vi "Modbus_Get_Temp.vi"(10 "register values":u16[](array[numeric]), 11 "Temp. unit:":u16) -> (2 "Numeric":dbl, 3 "Strings []":string[](array[string]))   [LabVIEW 2020]
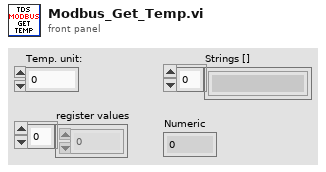
[diagram p1: front panel]
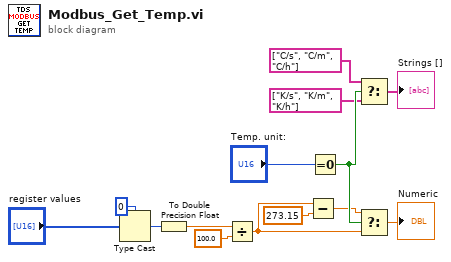
[diagram p0: block diagram]
diagram:
  n1 = Type Cast(type=0, x="register values") -> (*(type *) &x=w2:i32)
  n2 = To Double Precision Float(number=w2) -> (double precision float=w4:dbl)
  n3 = Divide(x=w4, y=100.0) -> (x/y=w6:dbl)
  n4 = Subtract(x=w6, y=273.15) -> (x-y=w8:dbl)
  n5 = Equal To 0?(x="Temp. unit:") -> (x = 0?=w13:bool)
  n6 = Select(t=string[] ["C/s", "C/m", "C/h"] ("Strings []"), s=w13, f=string[] ["K/s", "K/m", "K/h"] ("Strings []")) -> (s? t:f=→"Strings []":string[])
  n7 = Select(t=w8, s=w13, f=w6) -> (s? t:f=→"Numeric":dbl)
